vi "Edit Icon 2012.vi"(8 "error in (no error)":errorcluster, 10 "Color 256 in":T1={"image type"=0, "image depth"=24, "image"=array[3072 elements], "mask"=[], "colors"=[], "Rectangle"={"left"=0, "top"=0, "right"=32, "bottom"=32}}) -> (0 "error out":errorcluster, 2 "Color 256 out":T1)   [LabVIEW 2011]
uses:
  <vilib>/picture/picture.llb/imagedata.ctl
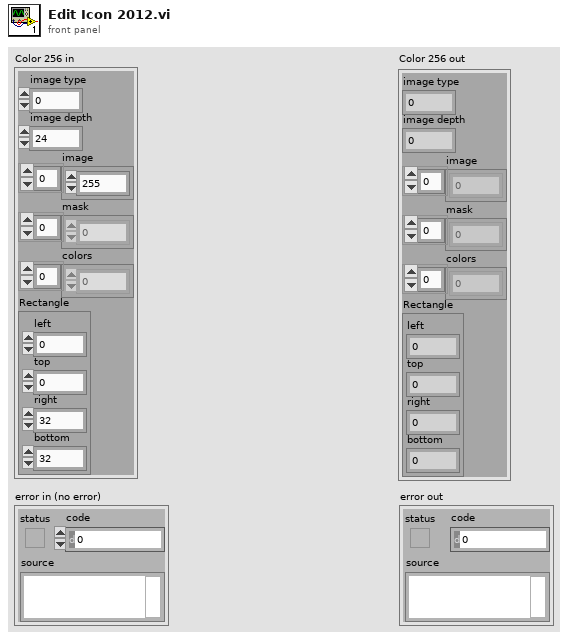
[diagram p1: front panel]
types:
  T1 = typedef "imagedata.ctl" = cluster{"image type":i32, "image depth":i32, "image":u8[], "mask":u8[], "colors":u32[], "Rectangle":cluster{"left":i16, "top":i16, "right":i16, "bottom":i16}}
  T2 = typedef "LabVIEW Icon Stored Information.ctl" = cluster{"Text Visible?":bool, "Text Opacity":u8, "Templ Visible?":bool, "Templ Opacity":u8, "Relative Path from 1 to 2":path, "Image":picture, "All User Layers":refnum<class "Layer.lvclass">[], "Body Text":T3}
  T3 = typedef "BodyText.ctl" = cluster{"Line 1 text":string, "Line 2 text":string, "Line 3 text":string, "Line 4 text":string, "Line 1 color":u32, "Line 2 color":u32, "Line 3 color":u32, "Line 4 color":u32, "Body Text Spec":cluster{"Font":T4, "Alignment":T5, "Size":u8}, "Center text vertically":bool, "Capitalize Text":bool}
  T4 = typedef "Font.ctl" = string
  T5 = typedef "Alignment.ctl" = u16
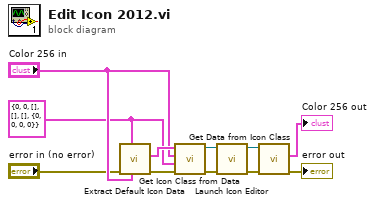
[diagram p0: block diagram]
diagram:
  w9 = T1 {"image type"=0, "image depth"=0, "image"=[], "mask"=[], "colors"=[], "Rectangle"={"left"=0, "top"=0, "right"=0, "bottom"=0}} ("BW Icon")
  n1 = call <vilib>:"Extract Default Icon Data.vi"("Color Icon"="Color 256 in", "BW Icon"=w9, "error in (no error)"="error in (no error)") -> ("error out"=w8:errorcluster, "VI Icon Data out"=w11:T2)  [unwired: 6 in, 1 out]
  n2 = call <vilib>:"Get Icon Class from Data.vi"("error in (no error)"=w8, "BW Icon"=w9, "Color Icon"="Color 256 in", "Icon Data"=w11) -> ("error out"=w6:errorcluster, "Icon out"=w7:refnum<class "Icon.lvclass">)  [unwired: 6 in]
  n3 = call <vilib>:"Launch Icon Editor.vi"("error in (no error)"=w6, "Icon in"=w7) -> ("error out"=w4:errorcluster, "Icon out"=w5:refnum<class "Icon.lvclass">)  [unwired: 7 in, 1 out]
  n4 = call <vilib>:"Get Data from Icon Class.vi"("error in (no error)"=w4, "Icon in"=w5) -> ("error out"=→"error out":errorcluster, "Color Image Data"=→"Color 256 out":T1)  [unwired: 6 in, 2 out]
